vi "PRN Generation.vi"(7 "FILE NAME":string="STATION1", 8 "error in (no error)":errorcluster, 9 "Cluster":T2, 10 "PRN path":path, 11 "File Folder Name":string="PSA") -> (0 "error out":errorcluster, 3 "PRN to Print":string, 4 "Barcode":string)   [LabVIEW 2017]
uses:
  <vilib>/addons/database/Connection.llb/Conn ObjectReference.ctl
  <vilib>/addons/database/NI_Database_API.lvlib
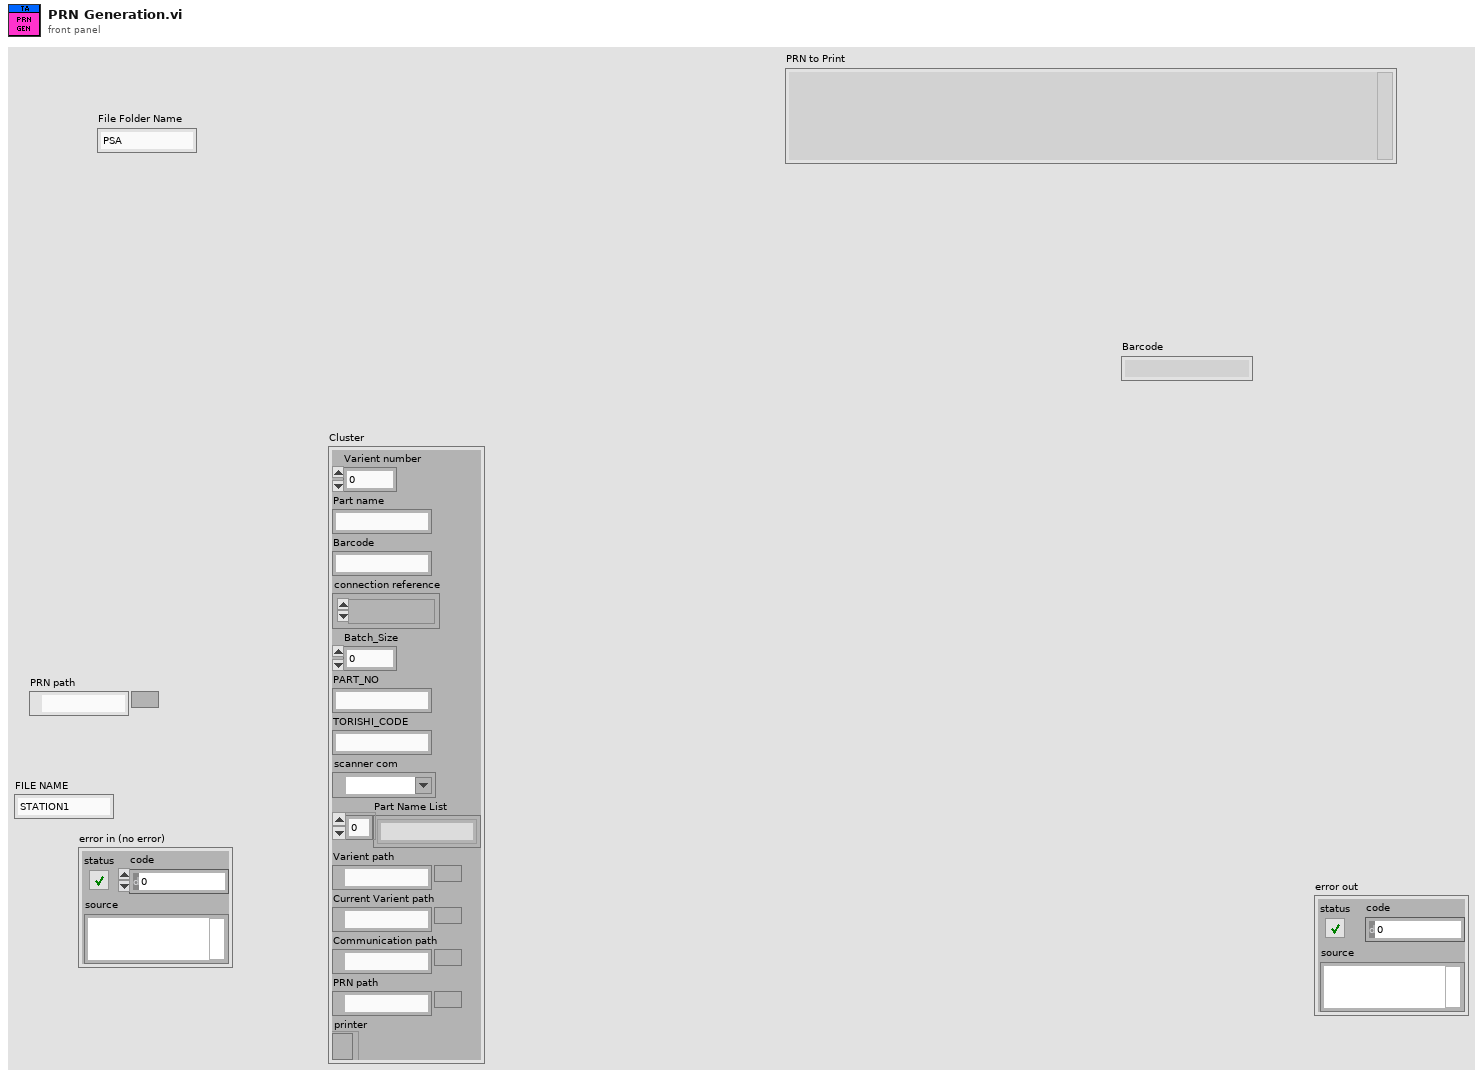
[diagram p1: front panel]
types:
  T1 = typedef "NI_Database_API.lvlib/Conn ObjectReference.ctl" = refnum<k1>
  T2 = cluster{"Varient number":u16, "Part name":string, "Barcode":string, "connection reference":T1, "Batch_Size":u16, "PART_NO":string, "TORISHI_CODE":string, "scanner com":refnum<visa-resource-name>, "Part Name List":string[], "Varient path":path, "Current Varient path":path, "Communication path":path, "PRN path":path, "printer":refnum<k5>}
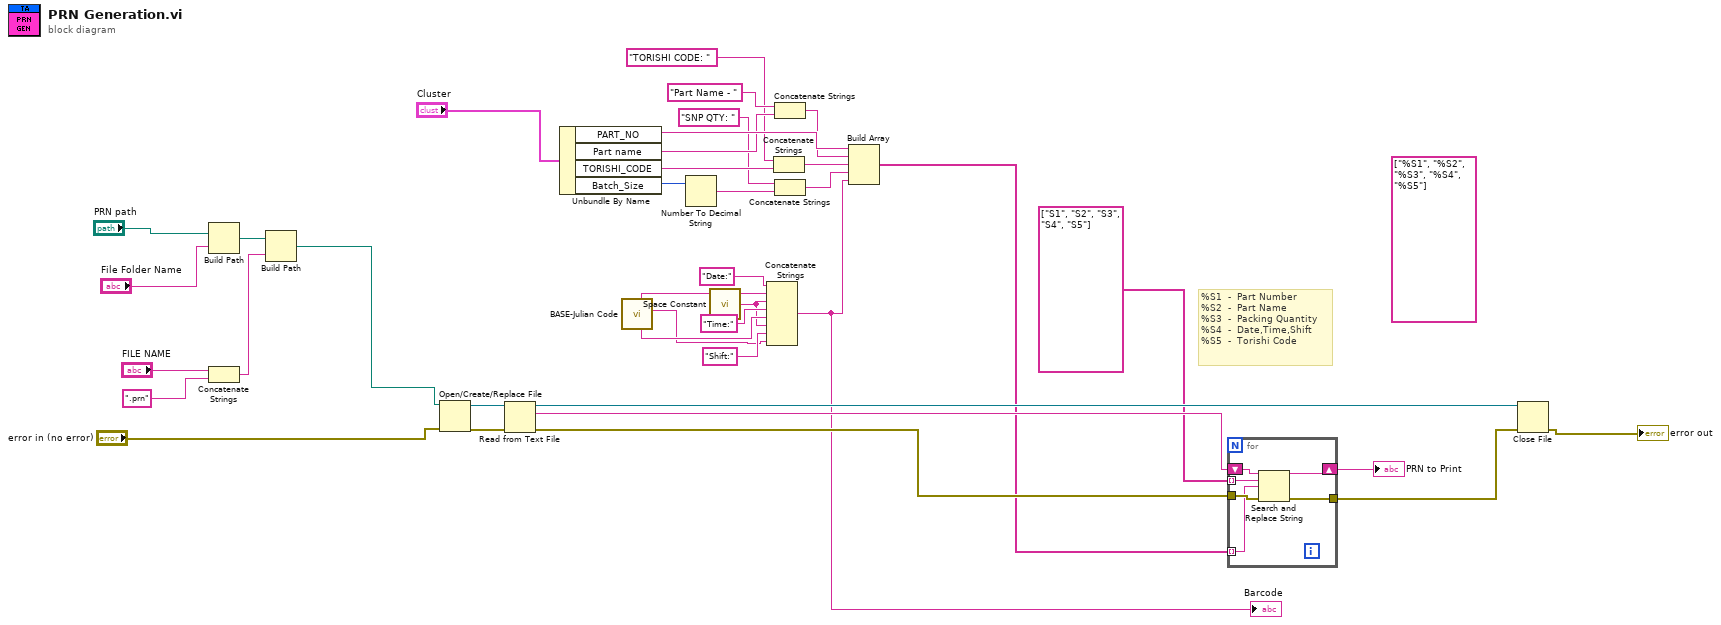
[diagram p0: block diagram]
diagram:
  (unwired) string[] ["%S1", "%S2", "%S3", "%S4", "%S5"]
  # "%S1  -  Part Number\n%S2  -  Part Name\n%S3  -  Packing Quantity\n%S4  -  Date,Time,Shift\n%S5  -  Torishi Code"
  n1 = Build Path(base path="PRN path", name or relative path="File Folder Name") -> (appended path=w26:path)
  n2 = Concatenate Strings("FILE NAME", ".prn" ("name or relative path")) -> (w28:string)
  n3 = Build Path(base path=w26, name or relative path=w28) -> (appended path=w23:path)
  n4 = Open/Create/Replace File(file path (use dialog)=w23, error in="error in (no error)") -> (refnum out=w35:refnum<file>, error out=w36:errorcluster)  [unwired: 4 in, 1 out]
  n5 = Read from Text File(file (use dialog)=w35, error in=w36) -> (refnum out=w37:refnum<file>, text=w33:string, error out=w31:errorcluster)  [unwired: 2 in, 1 out]
  n6 = Unbundle By Name("Cluster") -> ("PART_NO"=w20:string, "Part name"=w17:string, "TORISHI_CODE"=w15:string, "Batch_Size"=w21:u16)
  n7 = call "BASE-Julian Code.vi"() -> ("Shift"=w4:string, "Long time with :"=w7:string, "Long date with /"=w9:string)  [unwired: 6 in, 3 out]
  n8 = Number To Decimal String(number=w21) -> (decimal integer string=w12:string)  [unwired: 1 in]
  n9 = call <vilib>:"Space Constant.vi"() -> ("String"=w6:string)
  n10 = Concatenate Strings("Date:" ("string"), w9, w6, "Time:" ("string"), w7, w6, "Shift:" ("string"), w4) -> (w2:string)
  "Barcode" <- w2
  n11 = Concatenate Strings("TORISHI CODE: " ("string"), w15) -> (w14:string)
  n12 = Concatenate Strings("Part Name - " ("string"), w17) -> (w18:string)
  n13 = Concatenate Strings("SNP QTY: " ("string"), w12) -> (w11:string)
  n14 = Build Array(w20, w18, w14, w11, w2) -> (w3:string[])
  n15 = for {
    shift-right: [w43] -> w32
    shift-left: w33 -> [w44]
    tunnel: w31 -> [w42]
    tunnel: [w41] -> w30
    tunnel: string[] ["S1", "S2", "S3", "S4", "S5"] -> [w40] mode=indexing
    tunnel: w3 -> [w39] mode=indexing
    n16 = Search and Replace String(input string=w44, search string=w40, replace string=w39, error in=w42) -> (result string=w43:string, error out=w41:errorcluster)  [unwired: 4 in, 2 out]
  }
  "PRN to Print" <- w32
  n17 = Close File(refnum=w37, error in=w30) -> (error out=→"error out":errorcluster)  [unwired: 1 out]
